vi "COMP-TeleRead.vi"() -> ()   [LabVIEW 2017]
panel:
  in  "Port":u16=9000
  in  "Stop":bool
  out "Data Out":dbl[](array[numeric])
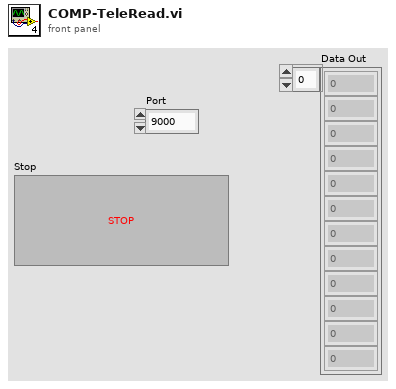
[diagram p1: front panel]
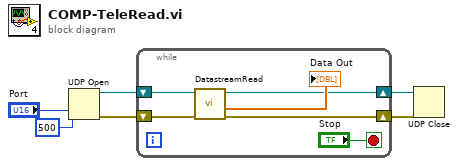
[diagram p0: block diagram]
diagram:
  n1 = UDP Open(9:500 ("timeout ms (25000)"), 11:"Port") -> (port=w6:refnum<k16>, 0:w5:errorcluster)  [unwired: 3 in, 1 out]
  n2 = while {
    shift-right: [w10] -> w2
    shift-left: w6 -> [w9]
    shift-right: [w7] -> w3
    shift-left: w5 -> [w8]
    stop <- "Stop" stop-if-true
    n3 = call "DatastreamRead.vi"("error in (no error)"=w8, "connection ID"=w9) -> ("error out"=w7:errorcluster, "Data Out"=→"Data Out":dbl[], "connection ID out"=w10:refnum<k16>)  [unwired: 7 in]
  }
  n4 = UDP Close(connection ID=w2, 8:w3) -> ()  [unwired: 2 out]
